vi "FLOM Pump Flow Write SubVI - standalone.vi"(0 "Write to Pump 1?":bool=TRUE, 1 "Write to Pump 2?":bool=TRUE, 2 "Mode":string(combo)="Continuous Flow", 3 "Edit Values, or Run Flow?\n(Only for Continuous Flow)":string(combo)="Run/Stop", 4 "Stop   Start":bool, 5 "Pump 1 Flow Rate (uL/min)":dbl=3000.0 min=0.0 max=9900.0 step=1.0, 6 "Stop   Start 2":bool, 7 "error in (no error) 2":errorcluster, 8 "Pump 2 Flow Rate (uL/min)":dbl=4000.0 min=0.0 max=9900.0 step=1.0, 9 "Data Cluster In":T1={"Flom Pump 1 Flow Rate"=0.0, "Script Running"=FALSE, "Unistat Set Temp"=0, "Flom Pump 2 Flow Rate"=0.0, "Flom Pump 1 Running"=FALSE, "Flom Pump 2 Running"=FALSE, "Unistat Running"=FALSE, "Line 1 Flow"=0.0, "Line 2 Flow"=0.0, "Product Temp"=0.0, "Product Flow"=0.0, "HEF Inlet"=0.0, "HEF Outlet"=0.0, "Line 1 Pressure"=0.0, "Line 2 Pressure"=0.0, "Line 3 Pressure"=0.0, "Pump 1 Pressure"=0.0, "Pump 2 Pressure"=0.0, "Number of Steps"=0.0, "Current Step Number"=0.0, "Pump 2 Flow Increment"=0.0, "Step Temp Increment"=0.0, "Step Function Start Time"=0.0, "Pump 2"=FALSE, "Pump 1"=TRUE, "Step Down?"=FALSE, "Number of Cycles"=0.0, "Pump 1 Initial Flow Rate"=0.0, "Pump 2 Initial Flow Rate"=0.0, "Initial Temperature"=0.0, "Step End Time"=0.0, "Pump 1 Current Step Flow"=0.0, "Pump 2 Current Step Flow"=0.0, "Current Step Temp"=0, "Time in each Step"=0.0, "Current Cycle Number"=0.0, "Turn off Temp after Step Flow?"=FALSE, "Internal Temp"=0.0, "Selected Path"=path "", "Excel Row Written"=0, "Counter at constant temp"=0.0, "Temp at Equilibrium"=FALSE, "Temp Equil Counter"=0.0, "Custom Step"=[{"Temp / C"=2, "Time / s"=0, "Flow 2 mL/m"=0.0, "Flow 1 mL/m"=0.0}, {"Temp / C"=2, "Time / s"=20, "Flow 2 mL/m"=0.0, "Flow 1 mL/m"=0.0}, {"Temp / C"=2, "Time / s"=100, "Flow 2 mL/m"=0.0, "Flow 1 mL/m"=0.0}, {"Temp / C"=2, "Time / s"=0, "Flow 2 mL/m"=0.0, "Flow 1 mL/m"=0.0}, {"Temp / C"=2, "Time / s"=90, "Flow 2 mL/m"=0.0, "Flow 1 mL/m"=0.0}, {"Temp / C"=2, "Time / s"=15, "Flow 2 mL/m"=0.0, "Flow 1 mL/m"=0.0}, {"Temp / C"=2, "Time / s"=0, "Flow 2 mL/m"=0.0, "Flow 1 mL/m"=0.0}, {"Temp / C"=2, "Time / s"=75, "Flow 2 mL/m"=0.0, "Flow 1 mL/m"=0.0}, {"Temp / C"=2, "Time / s"=2, "Flow 2 mL/m"=0.0, "Flow 1 mL/m"=0.0}], "Custom Step Number"=0.0, "Current Step t=0?"=FALSE, "Write to File"=FALSE, "Global Initialization Variables"={"Reactor Pressure Hard Upper Limit (bar)"=10.0, "Temp Hard Upper Limit (C)"=80.0, "Temp Hard Lower Limit (C)"=0.0, "Pump Minimum Flow (mL/min)"=0.0, "Pump Maximum Flow (mL/min)"=9.9, "Pump Interval (mL/min)"=0.001, "Temp Interval (C)"=0.1, "Flow Path Volume (mL)"=0.0}, "Error Message"="", "Program Error"=FALSE, "Pump Error"=FALSE, "Hardware Alert"=FALSE, "Comment"="", "Room Temp"=0.0, "VISA Resources"={"Flow VISA"="COM43", "Temp VISA"="COM43", "Flow VISA 1"="COM43", "Flow VISA 2"="COM43", "Flow VISA 3"="COM43", "Pressure VISA"="COM43", "Series IA VISA"="", "Series IB VISA"="", "Flow VISA 4"=""}, "Write Error"=FALSE, "Ports 1-5"=[FALSE, FALSE, FALSE, FALSE, FALSE, FALSE, FALSE, FALSE], "Pump 1 Flow Increment"=0.0, "Send to Product?"=FALSE, "Raman Spectrum Path"=path "", "Raman Spectrum Count"=0.0, "% Yield"=0.0, "Raman File Name"="", "New Spectrum?"=FALSE, "Last Spectrum Collected"=timestamp(0 s since 1904-01-01), "Line 4 Pressure"=0.0, "Series IA Pump Running"=FALSE, "Series IB Pump Running"=FALSE, "Series IA Pump Flow Rate"=0.0, "Series IB Pump Flow Rate"=0.0, "Line 3 Flow"=0.0, "Line 4 Flow"=0.0, "Series IA Pump Pressure"=0.0, "Series IB Pump Pressure"=0.0, "Flow Meter Cal Values"={"Flow Meter 2 Span Flow Rate"=10.0, "Flow Meter 1 Min Counts"=0.0, "Flow Meter 1 Max Counts"=9.9, "Flow Meter 1 Span Flow Rate"=0.01, "Flow Meter 2 Min Counts"=0.1, "Flow Meter 2 Max Counts"=0.0, "Flow Meter 4 Span Flow Rate"=10.0, "Flow Meter 3 Min Counts"=0.0, "Flow Meter 3 Max Counts"=9.9, "Flow Meter 3 Span Flow Rate"=0.01, "Flow Meter 4 Min Counts"=0.1, "Flow Meter 4 Max Counts"=0.0}, "Raman Exp?"=FALSE} {"Global Initialization Variables"."Reactor Pressure Hard Upper Limit (bar)" min=0.0 max=100.0 step=1.0}, 10 "Mode 2":string(combo)="Continuous Flow", 12 "Edit Values, or Run Flow?\n(Only for Continuous Flow) 2":string(combo)="Run/Stop", 15 "VISA resource":refnum<visa-resource-name>="COM8") -> (20 "Data Cluster Out":T1={"Flom Pump 1 Flow Rate"=0.0, "Script Running"=FALSE, "Unistat Set Temp"=0, "Flom Pump 2 Flow Rate"=0.0, "Flom Pump 1 Running"=FALSE, "Flom Pump 2 Running"=FALSE, "Unistat Running"=FALSE, "Line 1 Flow"=0.0, "Line 2 Flow"=0.0, "Product Temp"=0.0, "Product Flow"=0.0, "HEF Inlet"=0.0, "HEF Outlet"=0.0, "Line 1 Pressure"=0.0, "Line 2 Pressure"=0.0, "Line 3 Pressure"=0.0, "Pump 1 Pressure"=0.0, "Pump 2 Pressure"=0.0, "Number of Steps"=0.0, "Current Step Number"=0.0, "Pump 2 Flow Increment"=0.0, "Step Temp Increment"=0.0, "Step Function Start Time"=0.0, "Pump 2"=FALSE, "Pump 1"=TRUE, "Step Down?"=FALSE, "Number of Cycles"=0.0, "Pump 1 Initial Flow Rate"=0.0, "Pump 2 Initial Flow Rate"=0.0, "Initial Temperature"=0.0, "Step End Time"=0.0, "Pump 1 Current Step Flow"=0.0, "Pump 2 Current Step Flow"=0.0, "Current Step Temp"=0, "Time in each Step"=0.0, "Current Cycle Number"=0.0, "Turn off Temp after Step Flow?"=FALSE, "Internal Temp"=0.0, "Selected Path"=path "", "Excel Row Written"=0, "Counter at constant temp"=0.0, "Temp at Equilibrium"=FALSE, "Temp Equil Counter"=0.0, "Custom Step"=[{"Temp / C"=2, "Time / s"=0, "Flow 2 mL/m"=0.0, "Flow 1 mL/m"=0.0}, {"Temp / C"=2, "Time / s"=20, "Flow 2 mL/m"=0.0, "Flow 1 mL/m"=0.0}, {"Temp / C"=2, "Time / s"=100, "Flow 2 mL/m"=0.0, "Flow 1 mL/m"=0.0}, {"Temp / C"=2, "Time / s"=0, "Flow 2 mL/m"=0.0, "Flow 1 mL/m"=0.0}, {"Temp / C"=2, "Time / s"=90, "Flow 2 mL/m"=0.0, "Flow 1 mL/m"=0.0}, {"Temp / C"=2, "Time / s"=15, "Flow 2 mL/m"=0.0, "Flow 1 mL/m"=0.0}, {"Temp / C"=2, "Time / s"=0, "Flow 2 mL/m"=0.0, "Flow 1 mL/m"=0.0}, {"Temp / C"=2, "Time / s"=75, "Flow 2 mL/m"=0.0, "Flow 1 mL/m"=0.0}, {"Temp / C"=2, "Time / s"=2, "Flow 2 mL/m"=0.0, "Flow 1 mL/m"=0.0}], "Custom Step Number"=0.0, "Current Step t=0?"=FALSE, "Write to File"=FALSE, "Global Initialization Variables"={"Reactor Pressure Hard Upper Limit (bar)"=10.0, "Temp Hard Upper Limit (C)"=80.0, "Temp Hard Lower Limit (C)"=0.0, "Pump Minimum Flow (mL/min)"=0.0, "Pump Maximum Flow (mL/min)"=9.9, "Pump Interval (mL/min)"=0.001, "Temp Interval (C)"=0.1, "Flow Path Volume (mL)"=0.0}, "Error Message"="", "Program Error"=FALSE, "Pump Error"=FALSE, "Hardware Alert"=TRUE, "Comment"="", "Room Temp"=0.0, "VISA Resources"={"Flow VISA"="COM43", "Temp VISA"="COM43", "Flow VISA 1"="COM43", "Flow VISA 2"="COM43", "Flow VISA 3"="COM43", "Pressure VISA"="COM43", "Series IA VISA"="", "Series IB VISA"="", "Flow VISA 4"=""}, "Write Error"=FALSE, "Ports 1-5"=[FALSE, FALSE, FALSE, FALSE, FALSE, FALSE, FALSE, FALSE], "Pump 1 Flow Increment"=0.0, "Send to Product?"=FALSE, "Raman Spectrum Path"=path "", "Raman Spectrum Count"=0.0, "% Yield"=0.0, "Raman File Name"="", "New Spectrum?"=FALSE, "Last Spectrum Collected"=timestamp(0 s since 1904-01-01), "Line 4 Pressure"=0.0, "Series IA Pump Running"=FALSE, "Series IB Pump Running"=FALSE, "Series IA Pump Flow Rate"=0.0, "Series IB Pump Flow Rate"=0.0, "Line 3 Flow"=0.0, "Line 4 Flow"=0.0, "Series IA Pump Pressure"=0.0, "Series IB Pump Pressure"=0.0, "Flow Meter Cal Values"={"Flow Meter 2 Span Flow Rate"=10.0, "Flow Meter 1 Min Counts"=0.0, "Flow Meter 1 Max Counts"=9.9, "Flow Meter 1 Span Flow Rate"=0.01, "Flow Meter 2 Min Counts"=0.1, "Flow Meter 2 Max Counts"=0.0, "Flow Meter 4 Span Flow Rate"=10.0, "Flow Meter 3 Min Counts"=0.0, "Flow Meter 3 Max Counts"=9.9, "Flow Meter 3 Span Flow Rate"=0.01, "Flow Meter 4 Min Counts"=0.1, "Flow Meter 4 Max Counts"=0.0}, "Raman Exp?"=FALSE} {"Global Initialization Variables"."Reactor Pressure Hard Upper Limit (bar)" min=0.0 max=100.0 step=1.0}, 27 "Error Out":T2)   [LabVIEW 2015]
doc: "Written 12/2010 by Michael Roberto for control and monitoring of Flom high pressure liquid chromatography (HPLC) pumps.\n\nThis VI's purpose is to control the HPLC pumps, in conjunctiton with monitoring pressure and temperature in the reactor, and controlling the temperature via a heating system (yet to be integrated). To do this, the user first chooses the COM port in the VISA resource name box. Then pump number (set up seperately on the pump) is chosen. The user then chooses what kind of interaction they wish to perform with the pump: Continuous Flow, Step Flow, Status, or Reset. Discussion will focus mostly on Continuous and Step Flow commands.\n\nTo execute any command, the EXECUTE button must be pressed, to ensure that the commands are all set and that the pump receives the command only once.\n\nWhen using Continuous Flow, only use the drop down box labeled \"Only for Continuous Flow.\" Using the other boxes or numeric indicators when they're not specifically queried will not cause an error, but it's easier to understand when they're clear or, in the case of step number or time for continuous flow, zero. The flow rate for continuous flow is set seperately from the run/stop command. To edit the flow rate, choose \"edit\" from the drop-down menu and enter a flow rate in the Flow Rate box. Press the EXECUTE button to send the command to the pump. To begin flow, choose \"Start/Stop\" from the drop-down box, and set the switch into the \"Start\" position, and press the EXECUTE button. To stop, switch to Stop and press EXECUTE.\nIn continuous flow, flow rate can be changed while the pump is flowing. Same as before, choose \"edit,\" enter the flow rate, and press EXECUTE.\n\nStep mode is more complicated to run, as flow rates need to be established for each step separately, and the initial flow rate must stipulate how many steps will be executed. I hope to write a VI in the future that, when given a command such as \"20 steps, 0.1 ul/min increments, for 20 minutes,\" will go through and perform these itself, but for now they each have to be performed separately.\n\nGeneric Step Instructions: \nFirst, set up an initial flow rate by choosing such in the drop down menu. It's *important* that you dictate how many steps will be in the program as well. It must be chosen before you hit EXECUTE when setting the initial flow rate.\nSecond, you must define the flow rate and time and step method (linear vs. step) for each step, in the 'configure step' drop down menu. So you would set the step at \"1\", flow rate at the desired flow, and for the desired time length, then press EXECUTE. Then change all those variables again for the 2nd step, and so on. The pump will not recognize commands if you exceed the number of steps dictated in the initial flow rate.\nThird, you run the initial flow rate, by choosing so from the drop down menu and pressing EXECUTE when the switch is in the Start position\nFourth, run the step program.\nAfter the Step Program has finished, the pump will return to the initial flow rate, and will not turn off until you switch to \"Stop\" while in the \"Run initial flow rate\" drop down and hitting EXECUTE."
uses:
  --Controls and TypeDefs--/Control_LDH.ctl
  <vilib>/Instr/_visa.llb/VISA Configure Serial Port (Instr).vi
panel:
  in  "Step   Linear 2":bool
  in  "Step Flow Commands \n(Only For Step Flow) 2":string(combo)
  in  "Time (.01 mins) 2":i32 min=0 max=9999 step=1
  in  "Step # 2":i32 min=0 max=49 step=1
  in  "Setup Commands\n(Only for Setup) 2":string(combo)
  in  "Request Commands\n(Only for Status) 2":string(combo)
  in  "Step   Linear":bool
  out "String to Write to Pump 2":string="P2,G1,0"
  in  "bytes to read 2":u32=40
  out "actual bytes read 2":u32=9
  out "P2 Flowing?":bool
  out "Last message received from Pump 2":string="Pump 2 message, 10:06:19 AM:\nProgram Error: Prohibited command (conflicting operation command)"
  out "Status of Pump 2":string
  out "P1 Flowing?":bool
  out "Last message received from Pump 1":string="Pump 1 message, 10:06:19 AM:\nProgram Error: Prohibited command (conflicting operation command)"
  in  "Step Flow Commands \n(Only For Step Flow)":string(combo)
  in  "Time (.01 mins)":i32 min=0 max=9999 step=1
  in  "Step #":i32 min=0 max=49 step=1
  in  "Setup Commands\n(Only for Setup)":string(combo)
  in  "Request Commands\n(Only for Status)":string(combo)
  out "String to Write to Pump 1":string="P1,G1,0"
  out "actual bytes read":u32=8
  in  "bytes to read":u32=40
  out "Status of Pump 1":string
  # "Flom Pump Control VI.  Continuously queries status of pump, writes to pump with \"EXECUTE\" button press."
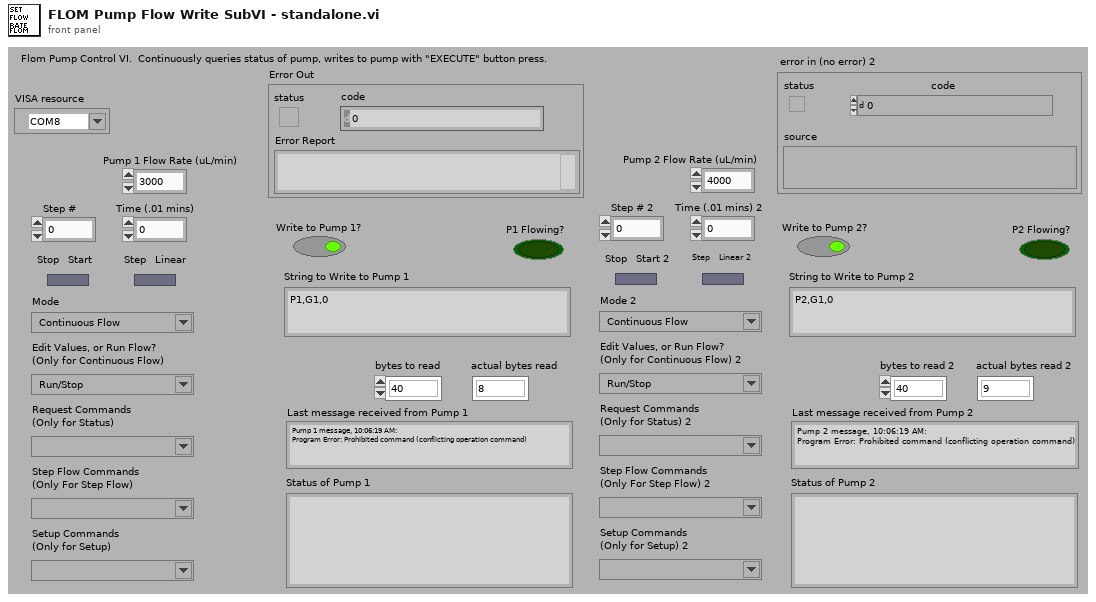
[diagram p1: front panel]
types:
  T1 = typedef "Control_LDH.ctl" = cluster{"Flom Pump 1 Flow Rate":dbl, "Script Running":bool, "Unistat Set Temp":i32, "Flom Pump 2 Flow Rate":dbl, "Flom Pump 1 Running":bool, "Flom Pump 2 Running":bool, "Unistat Running":bool, "Line 1 Flow":dbl, "Line 2 Flow":dbl, "Product Temp":dbl, "Product Flow":dbl, "HEF Inlet":dbl, "HEF Outlet":dbl, "Line 1 Pressure":dbl, "Line 2 Pressure":dbl, "Line 3 Pressure":dbl, "Pump 1 Pressure":dbl, "Pump 2 Pressure":dbl, "Number of Steps":dbl, "Current Step Number":dbl, "Pump 2 Flow Increment":dbl, "Step Temp Increment":dbl, "Step Function Start Time":dbl, "Pump 2":bool, "Pump 1":bool, "Step Down?":bool, "Number of Cycles":dbl, "Pump 1 Initial Flow Rate":dbl, "Pump 2 Initial Flow Rate":dbl, "Initial Temperature":dbl, "Step End Time":dbl, "Pump 1 Current Step Flow":dbl, "Pump 2 Current Step Flow":dbl, "Current Step Temp":i32, "Time in each Step":dbl, "Current Cycle Number":dbl, "Turn off Temp after Step Flow?":bool, "Internal Temp":dbl, "Selected Path":path, "Excel Row Written":i32, "Counter at constant temp":dbl, "Temp at Equilibrium":bool, "Temp Equil Counter":dbl, "Custom Step":cluster{"Temp / C":u16, "Time / s":i32, "Flow 2 mL/m":dbl, "Flow 1 mL/m":dbl}[], "Custom Step Number":dbl, "Current Step t=0?":bool, "Write to File":bool, "Global Initialization Variables":cluster{"Reactor Pressure Hard Upper Limit (bar)":dbl, "Temp Hard Upper Limit (C)":dbl, "Temp Hard Lower Limit (C)":dbl, "Pump Minimum Flow (mL/min)":dbl, "Pump Maximum Flow (mL/min)":dbl, "Pump Interval (mL/min)":dbl, "Temp Interval (C)":dbl, "Flow Path Volume (mL)":dbl}, "Error Message":string, "Program Error":bool, "Pump Error":bool, "Hardware Alert":bool, "Comment":string, "Room Temp":dbl, "VISA Resources":cluster{"Flow VISA":refnum<visa-resource-name>, "Temp VISA":refnum<visa-resource-name>, "Flow VISA 1":refnum<visa-resource-name>, "Flow VISA 2":refnum<visa-resource-name>, "Flow VISA 3":refnum<visa-resource-name>, "Pressure VISA":refnum<visa-resource-name>, "Series IA VISA":refnum<visa-resource-name>, "Series IB VISA":refnum<visa-resource-name>, "Flow VISA 4":refnum<visa-resource-name>}, "Write Error":bool, "Ports 1-5":bool[], "Pump 1 Flow Increment":dbl, "Send to Product?":bool, "Raman Spectrum Path":path, "Raman Spectrum Count":dbl, "% Yield":dbl, "Raman File Name":string, "New Spectrum?":bool, "Last Spectrum Collected":timestamp, "Line 4 Pressure":dbl, "Series IA Pump Running":bool, "Series IB Pump Running":bool, "Series IA Pump Flow Rate":dbl, "Series IB Pump Flow Rate":dbl, "Line 3 Flow":dbl, "Line 4 Flow":dbl, "Series IA Pump Pressure":dbl, "Series IB Pump Pressure":dbl, "Flow Meter Cal Values":cluster{"Flow Meter 2 Span Flow Rate":dbl, "Flow Meter 1 Min Counts":dbl, "Flow Meter 1 Max Counts":dbl, "Flow Meter 1 Span Flow Rate":dbl, "Flow Meter 2 Min Counts":dbl, "Flow Meter 2 Max Counts":dbl, "Flow Meter 4 Span Flow Rate":dbl, "Flow Meter 3 Min Counts":dbl, "Flow Meter 3 Max Counts":dbl, "Flow Meter 3 Span Flow Rate":dbl, "Flow Meter 4 Min Counts":dbl, "Flow Meter 4 Max Counts":dbl}, "Raman Exp?":bool}
  T2 = cluster{"status":bool, "code":i32, "Error Report":string}
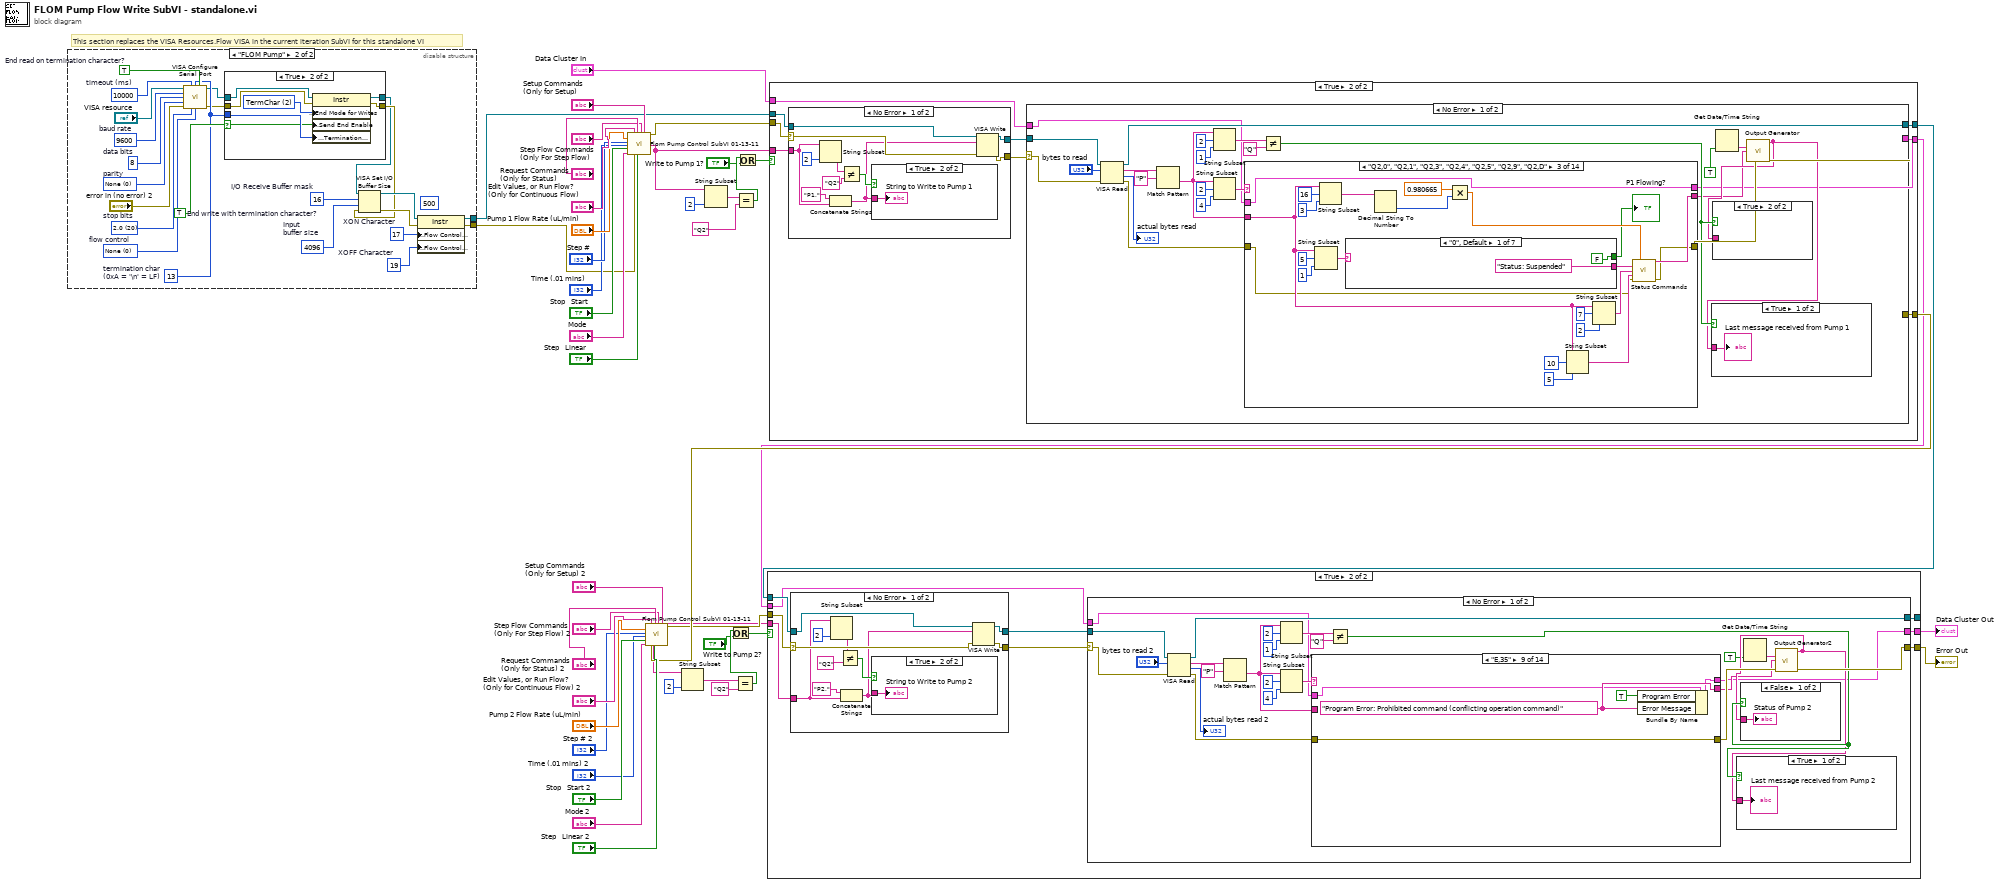
[diagram p0: block diagram]
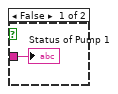
[diagram p5: hidden frame]
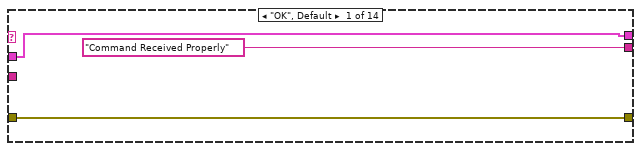
[diagram p7: hidden frame]
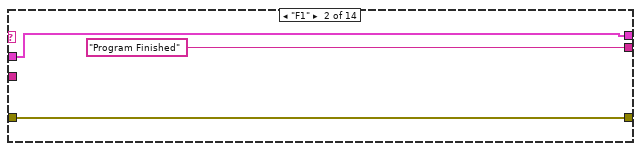
[diagram p8: hidden frame]
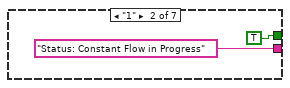
[diagram p9: hidden frame]
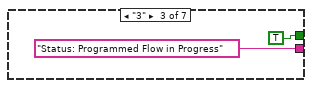
[diagram p10: hidden frame]
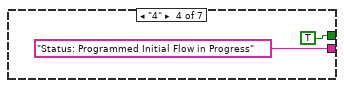
[diagram p11: hidden frame]
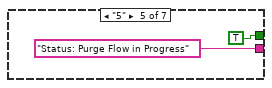
[diagram p12: hidden frame]
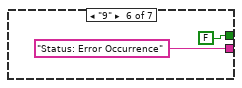
[diagram p13: hidden frame]
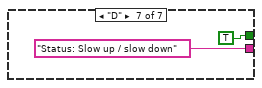
[diagram p14: hidden frame]
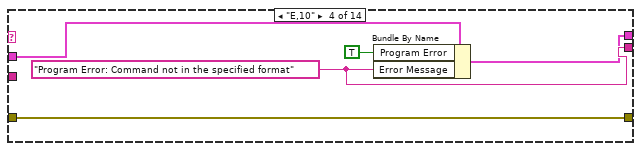
[diagram p15: hidden frame]
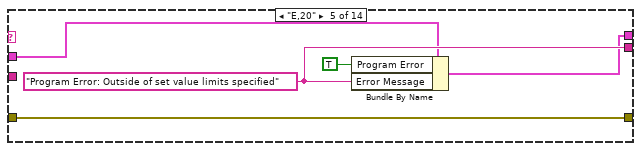
[diagram p16: hidden frame]
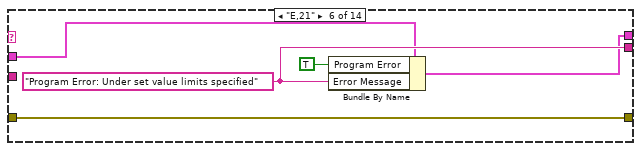
[diagram p17: hidden frame]
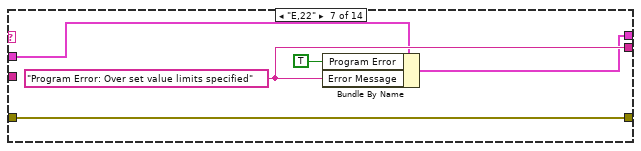
[diagram p18: hidden frame]
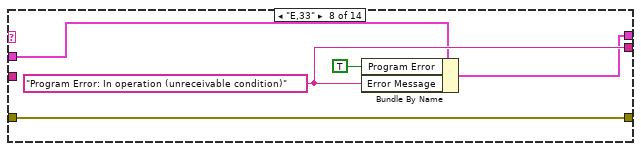
[diagram p19: hidden frame]
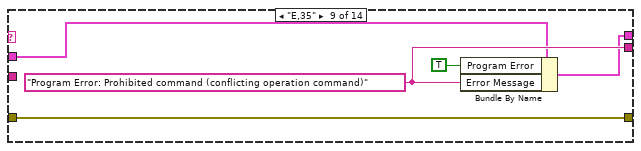
[diagram p20: hidden frame]
diagram:
  # "This section replaces the VISA Resources.Flow VISA in the current iteration SubVI for this standalone VI"
  n1 = disable-structure shown="\"FLOM Pump\"" {
    disable-tunnel: [_ w47] -> w2
    disable-tunnel: [_ w46] -> w1
    frame condition #0 {
    }
    frame condition #1 (active) {
      (unwired) 500
      w60 = u32 4096  # Input buffer size
      w53 = u8 19  # XOFF Character
      w54 = u8 17  # XON Character
      w63 = u32 10000  # timeout (ms)
      w62 = TRUE  # End read on termination character?
      w59 = TRUE  # End write with termination character?
      w58 = u8 13  # termination char (0xA = '\n' = LF)
      w57 = u16 0 items=["None"=0, "XON/XOFF"=1, "RTS/CTS"=2, "DTR/DSR"=4]  # flow control
      w64 = u16 20 items=["1.0"=10, "1.5"=15, "2.0"=20]  # stop bits
      w65 = u16 0 items=["None", "Odd", "Even", "Mark", "Space"]  # parity
      w52 = u16 8  # data bits
      w67 = u32 9600  # baud rate
      w61 = u16 16  # I/O Receive Buffer mask
      n2 = call-poly "VISA Configure Serial Port"("VISA resource name"="VISA resource", "timeout (10sec)"=w63, "termination char\n(0xA = '\\n' = LF)"=w58, "Enable Termination\nChar (T)"=w62, "baud rate (9600)"=w67, "data bits (8)"=w52, "parity (0:none)"=w65, "error in (no error)"="error in (no error) 2", "stop bits (10: 1 bit)"=w64, "flow control (0:none)"=w57) -> ("VISA resource name out"=w48:refnum<visa-resource-name>, "error out"=w51:errorcluster)  [unwired: 4 out]
      n3 = case shown="True" w59 {
        selector: w59 -> [_ w70]
        tunnel: w48 -> [w68 w76]
        tunnel: w51 -> [w69 w75]
        tunnel: [w68 w74] -> w49
        tunnel: [w69 w73] -> w50
        tunnel: w58 -> [_ w71]
        frame False {
        }
        frame True {
          w72 = u16 2 items=["None", "LastBit", "TermChar", "Break"] ("Serial Settings:Serial End Mode for Writes")
          n4 = property class="Instr"(reference=w76, error in=w75, "Serial Settings:End Mode for Writes"=w72, "Message Based Settings:Send End Enable"=w70, "Message Based Settings:Termination Character"=w71) -> (reference out=w74:refnum<visa-resource-name>, error out=w73:errorcluster)
        }
      }
      n5 = VISA Set I/O Buffer Size(VISA resource name=w49, mask (16)=w61, size (4096)=w60, error in (no error)=w50) -> (VISA resource name out=w56:refnum<visa-resource-name>, error out=w55:errorcluster)
      n6 = property class="Instr"(reference=w56, error in=w55, "Serial Settings:Flow Control XON Character"=w54, "Serial Settings:Flow Control XOFF Character"=w53) -> (reference out=w46:refnum<visa-resource-name>, error out=w47:errorcluster)
    }
  }
  n7 = call "Flom Pump Control SubVI 01-13-11.vi"("Flow Rate (uL)"="Pump 1 Flow Rate (uL/min)", "Step #"="Step #", "Time (.01 mins)"="Time (.01 mins)", "Stop   Start"="Stop   Start", "Mode"="Mode", "Edit Values, or Run Flow?\n(Only for Continuous Flow)"="Edit Values, or Run Flow?\n(Only for Continuous Flow)", "error in (no error)"=w2, "Request Commands\n(Only for Status)"="Request Commands\n(Only for Status)", "Step Linear"="Step   Linear", "Step Flow Commands \n(Only For Step Flow)"="Step Flow Commands \n(Only For Step Flow)", "Setup Commands\n(Only for Setup)"="Setup Commands\n(Only for Setup)") -> ("error out"=w4:errorcluster, "String"=w40:string)  [unwired: 1 in, 6 out]
  n8 = String Subset(string=w40, length (rest)=2) -> (substring=w42:string)  [unwired: 1 out]
  n9 = Equal?(x=w42, y="Q2") -> (x = y?=w39:bool)
  n10 = Or(x=w39, y="Write to Pump 1?") -> (x .or. y?=w37:bool)
  n11 = case shown="True" w37 {
    tunnel: w1 -> [w79 w86]
    tunnel: w4 -> [w78 w85]
    tunnel: [w79 w84] -> w44
    tunnel: [w78 w83] -> w10
    tunnel: w40 -> [_ w82]
    tunnel: "Data Cluster In" -> [w77 w81]
    tunnel: [w77 w80] -> w7
    frame False {
    }
    frame True {
      n12 = case shown="No Error" w85 {
        selector: w85 -> [w223 w229]
        tunnel: [w226 w228] -> w88
        tunnel: [w225 w229] -> w87
        tunnel: w86 -> [w224 w228]
        tunnel: w82 -> [w217 _]
        frame No Error {
          n13 = String Subset(string=w217, length (rest)=2) -> (substring=w220:string)  [unwired: 1 out]
          n14 = Concatenate Strings("P1,", w217) -> (w216:string)
          n15 = Not Equal?(x=w220, y="Q2") -> (x != y?=w218:bool)
          n16 = case shown="True" w218 {
            tunnel: w216 -> [_ w227]
            frame False {
            }
            frame True {
              "String to Write to Pump 1" <- w227
            }
          }
          n17 = VISA Write(VISA resource name=w224, write buffer=w216, error in (no error)=w223) -> (VISA resource name out=w226:refnum<visa-resource-name>, error out=w225:errorcluster)  [unwired: 1 out]
        }
        frame Error {
        }
      }
      n18 = case "Read bytes from port." shown="No Error" w87 {
        selector: w87 -> [w110 w214]
        tunnel: [w97 w214] -> w83
        tunnel: [w113 w215] -> w84
        tunnel: w88 -> [w111 w215]
        tunnel: w81 -> [w90 w213]
        tunnel: [w89 w213] -> w80
        frame No Error {
          n19 = VISA Read(VISA resource name=w111, byte count="bytes to read", error in (no error)=w110) -> (VISA resource name out=w113:refnum<visa-resource-name>, read buffer=w104:string, return count=→"actual bytes read":u32, error out=w99:errorcluster)
          n20 = Match Pattern(string=w104, regular expression="P") -> (after substring=w96:string)  [unwired: 4 out]
          n21 = String Subset(string=w96, offset (0)=2, length (rest)=1) -> (substring=w101:string)
          n22 = String Subset(string=w96, offset (0)=2, length (rest)=4) -> (substring=w108:string)
          n23 = case shown="\"Q2,0\", \"Q2,1\", \"Q2,3\", \"Q2,4\", \"Q2,5\", \"Q2,9\", \"Q2,D\"" w108 {
            tunnel: ["Command Received Properly" "Program Finished" w128 w159 w165 w170 w175 w180 w185 w190 w195 w200 w205 w210] -> w91
            tunnel: w96 -> [_ _ w126 _ _ _ _ _ _ _ _ _ _ _]
            tunnel: w99 -> [w117 w120 w125 w162 w167 w172 w177 w182 w187 w192 w197 w202 w207 w212]
            tunnel: [w117 w120 w124 w162 w167 w172 w177 w182 w187 w192 w197 w202 w207 w212] -> w98
            tunnel: w90 -> [w116 w119 w122 w161 w164 w168 w174 w179 w184 w189 w194 w199 w204 w209]
            tunnel: [w116 w119 w122 w158 w163 w169 w173 w178 w183 w188 w193 w198 w203 w208] -> w89
            frame "OK", Default {
            }
            frame "F1" {
            }
            frame "Q2,0", "Q2,1", "Q2,3", "Q2,4", "Q2,5", "Q2,9", "Q2,D" {
              n24 = String Subset(string=w126, offset (0)=5, length (rest)=1) -> (substring=w127:string)
              n25 = String Subset(string=w126, offset (0)=16, length (rest)=3) -> (substring=w135:string)
              n26 = case shown="\"0\", Default" w127 {
                tunnel: ["Status: Suspended" "Status: Constant Flow in Progress" "Status: Programmed Flow in Progress" "Status: Programmed Initial Flow in Progress" "Status: Purge Flow in Progress" "Status: Error Occurrence" "Status: Slow up / slow down"] -> w132
                tunnel: [FALSE TRUE TRUE TRUE TRUE FALSE TRUE] -> w123
                frame "0", Default {
                }
                frame "1" {
                }
                frame "3" {
                }
                frame "4" {
                }
                frame "5" {
                }
                frame "9" {
                }
                frame "D" {
                }
              }
              "P1 Flowing?" <- w123
              n27 = Decimal String To Number(string=w135) -> (number=w134:i32)  [unwired: 3 out]
              n28 = Multiply(x=0.980665, y=w134) -> (x*y=w129:dbl)
              n29 = String Subset(string=w126, offset (0)=10, length (rest)=5) -> (substring=w130:string)
              n30 = String Subset(string=w126, offset (0)=7, length (rest)=2) -> (substring=w131:string)
              n31 = call "Status Commands"("press"=w129, "Status"=w132, "step num"=w131, "flow"=w130, "error in (no error)"=w125) -> ("Result"=w128:string, "error out"=w124:errorcluster)  [unwired: 1 in, 8 out]
            }
            frame "E,10" {
              w159 = "Program Error: Command not in the specified format"
              n32 = Bundle By Name(cluster=w161, "Program Error"=TRUE, "Error Message"=w159) -> (w158:T1)
            }
            frame "E,20" {
              w165 = "Program Error: Outside of set value limits specified"
              n33 = Bundle By Name(cluster=w164, "Program Error"=TRUE, "Error Message"=w165) -> (w163:T1)
            }
            frame "E,21" {
              w170 = "Program Error: Under set value limits specified"
              n34 = Bundle By Name(cluster=w168, "Program Error"=TRUE, "Error Message"=w170) -> (w169:T1)
            }
            frame "E,22" {
              w175 = "Program Error: Over set value limits specified"
              n35 = Bundle By Name(cluster=w174, "Program Error"=TRUE, "Error Message"=w175) -> (w173:T1)
            }
            frame "E,33" {
              w180 = "Program Error: In operation (unreceivable condition)"
              n36 = Bundle By Name(cluster=w179, "Program Error"=TRUE, "Error Message"=w180) -> (w178:T1)
            }
            frame "E,35" {
              w185 = "Program Error: Prohibited command (conflicting operation command)"
              n37 = Bundle By Name(cluster=w184, "Program Error"=TRUE, "Error Message"=w185) -> (w183:T1)
            }
            frame "E,52" {
              w190 = "Program Error: Error due to unconnected subordinate pumps (CTS error)"
              n38 = Bundle By Name(cluster=w189, "Program Error"=TRUE, "Error Message"=w190) -> (w188:T1)
            }
            frame "E,61" {
              w195 = "Pump Error: Error after the upper pressure limit is exceeded"
              n39 = Bundle By Name(cluster=w194, "Pump Error"=TRUE, "Error Message"=w195) -> (w193:T1)
            }
            frame "E,62" {
              w200 = "Pump Error: Error after the lower pressure limit is exceeded"
              n40 = Bundle By Name(cluster=w199, "Pump Error"=TRUE, "Error Message"=w200) -> (w198:T1)
            }
            frame "E,63" {
              w205 = "Pump Error: Check-valve error"
              n41 = Bundle By Name(cluster=w204, "Pump Error"=TRUE, "Error Message"=w205) -> (w203:T1)
            }
            frame "E,64" {
              w210 = "Pump Error: Irregular Rotation Error"
              n42 = Bundle By Name(cluster=w209, "Pump Error"=TRUE, "Error Message"=w210) -> (w208:T1)
            }
          }
          n43 = Not Equal?(x=w101, y="Q") -> (x != y?=w95:bool)
          n44 = Get Date/Time String(want seconds? (F)=TRUE) -> (time string=w92:string)  [unwired: 3 out]
          n45 = call "Output Generator"("Time"=w92, "Error Output"=w91, "error in (no error)"=w98) -> ("Result"=w94:string, "error out"=w97:errorcluster)  [unwired: 2 in, 9 out]
          n46 = case shown="True" w95 {
            tunnel: w94 -> [w115 _]
            frame True {
              "Last message received from Pump 1" <- w115
            }
            frame False {
            }
          }
          n47 = case shown="True" w95 {
            tunnel: w94 -> [w114 _]
            frame False {
              "Status of Pump 1" <- w114
            }
            frame True {
            }
          }
        }
        frame Error {
        }
      }
    }
  }
  n48 = call "Flom Pump Control SubVI 01-13-11.vi"("Flow Rate (uL)"="Pump 2 Flow Rate (uL/min)", "Step #"="Step # 2", "Time (.01 mins)"="Time (.01 mins) 2", "Stop   Start"="Stop   Start 2", "Mode"="Mode 2", "Edit Values, or Run Flow?\n(Only for Continuous Flow)"="Edit Values, or Run Flow?\n(Only for Continuous Flow) 2", "error in (no error)"=w10, "Request Commands\n(Only for Status)"="Request Commands\n(Only for Status) 2", "Step Linear"="Step   Linear 2", "Step Flow Commands \n(Only For Step Flow)"="Step Flow Commands \n(Only For Step Flow) 2", "Setup Commands\n(Only for Setup)"="Setup Commands\n(Only for Setup) 2") -> ("error out"=w9:errorcluster, "String"=w8:string)  [unwired: 1 in, 6 out]
  n49 = String Subset(string=w8, length (rest)=2) -> (substring=w35:string)  [unwired: 1 out]
  n50 = Equal?(x=w35, y="Q2") -> (x = y?=w33:bool)
  n51 = Or(x=w33, y="Write to Pump 2?") -> (x .or. y?=w31:bool)
  n52 = case shown="True" w31 {
    tunnel: [w231 w239] -> w3
    tunnel: [w232 w238] -> _
    tunnel: w44 -> [w232 w237]
    tunnel: w9 -> [w231 w236]
    tunnel: w8 -> [_ w235]
    tunnel: w7 -> [w230 w234]
    tunnel: [w230 w233] -> w6
    frame False {
    }
    frame True {
      n53 = case shown="No Error" w236 {
        selector: w236 -> [w249 w255]
        tunnel: [w252 w254] -> w241
        tunnel: [w251 w255] -> w240
        tunnel: w237 -> [w250 w254]
        tunnel: w235 -> [w242 _]
        frame No Error {
          n54 = String Subset(string=w242, length (rest)=2) -> (substring=w246:string)  [unwired: 1 out]
          n55 = Not Equal?(x=w246, y="Q2") -> (x != y?=w244:bool)
          n56 = Concatenate Strings("P2,", w242) -> (w243:string)
          n57 = case shown="True" w244 {
            tunnel: w243 -> [_ w253]
            frame False {
            }
            frame True {
              "String to Write to Pump 2" <- w253
            }
          }
          n58 = VISA Write(VISA resource name=w250, write buffer=w243, error in (no error)=w249) -> (VISA resource name out=w252:refnum<visa-resource-name>, error out=w251:errorcluster)  [unwired: 1 out]
        }
        frame Error {
        }
      }
      n59 = case "Read bytes from port." shown="No Error" w240 {
        selector: w240 -> [w277 w381]
        tunnel: [w264 w381] -> w239
        tunnel: [w280 w382] -> w238
        tunnel: w241 -> [w278 w382]
        tunnel: w234 -> [w257 w380]
        tunnel: [w256 w380] -> w233
        frame No Error {
          n60 = VISA Read(VISA resource name=w278, byte count="bytes to read 2", error in (no error)=w277) -> (VISA resource name out=w280:refnum<visa-resource-name>, read buffer=w271:string, return count=→"actual bytes read 2":u32, error out=w266:errorcluster)
          n61 = Match Pattern(string=w271, regular expression="P") -> (after substring=w263:string)  [unwired: 4 out]
          n62 = String Subset(string=w263, offset (0)=2, length (rest)=1) -> (substring=w268:string)
          n63 = String Subset(string=w263, offset (0)=2, length (rest)=4) -> (substring=w275:string)
          n64 = case shown="\"E,35\"" w275 {
            tunnel: ["Command Received Properly" "Program Finished" w295 w327 w332 w337 w341 w347 w352 w356 w360 w367 w372 w377] -> w258
            tunnel: w263 -> [_ _ w293 _ _ _ _ _ _ _ _ _ _ _]
            tunnel: w266 -> [w284 w287 w292 w329 w334 w339 w344 w349 w354 w359 w364 w369 w374 w379]
            tunnel: [w284 w287 w291 w329 w334 w339 w344 w349 w354 w359 w364 w369 w374 w379] -> w265
            tunnel: w257 -> [w283 w286 w289 w326 w331 w336 w342 w346 w351 w357 w362 w366 w371 w376]
            tunnel: [w283 w286 w289 w325 w330 w335 w340 w345 w350 w355 w361 w365 w370 w375] -> w256
            frame "OK", Default {
            }
            frame "F1" {
            }
            frame "Q2,0", "Q2,1", "Q2,3", "Q2,4", "Q2,5", "Q2,9", "Q2,D" {
              n65 = String Subset(string=w293, offset (0)=5, length (rest)=1) -> (substring=w294:string)
              n66 = String Subset(string=w293, offset (0)=16, length (rest)=3) -> (substring=w302:string)
              n67 = case shown="\"4\"" w294 {
                tunnel: ["Status: Suspended" "Status: Constant Flow in Progress" "Status: Programmed Flow in Progress" "Status: Programmed Initial Flow in Progress" "Status: Purge Flow in Progress" "Status: Error Occurrence" "Status: Slow up / slow down"] -> w299
                tunnel: [FALSE TRUE TRUE TRUE TRUE FALSE TRUE] -> w290
                frame "0", Default {
                }
                frame "1" {
                }
                frame "3" {
                }
                frame "4" {
                }
                frame "5" {
                }
                frame "9" {
                }
                frame "D" {
                }
              }
              "P2 Flowing?" <- w290
              n68 = Decimal String To Number(string=w302) -> (number=w301:i32)  [unwired: 3 out]
              n69 = String Subset(string=w293, offset (0)=10, length (rest)=5) -> (substring=w297:string)
              n70 = Multiply(x=0.980665, y=w301) -> (x*y=w296:dbl)
              n71 = String Subset(string=w293, offset (0)=7, length (rest)=2) -> (substring=w298:string)
              n72 = call "Status Commands2"("press"=w296, "Status"=w299, "step num"=w298, "flow"=w297, "error in (no error)"=w292) -> ("Result"=w295:string, "error out"=w291:errorcluster)  [unwired: 1 in, 8 out]
            }
            frame "E,10" {
              w327 = "Program Error: Command not in the specified format"
              n73 = Bundle By Name(cluster=w326, "Program Error"=TRUE, "Error Message"=w327) -> (w325:T1)
            }
            frame "E,20" {
              w332 = "Program Error: Outside of set value limits specified"
              n74 = Bundle By Name(cluster=w331, "Program Error"=TRUE, "Error Message"=w332) -> (w330:T1)
            }
            frame "E,21" {
              w337 = "Program Error: Under set value limits specified"
              n75 = Bundle By Name(cluster=w336, "Program Error"=TRUE, "Error Message"=w337) -> (w335:T1)
            }
            frame "E,22" {
              w341 = "Program Error: Over set value limits specified"
              n76 = Bundle By Name(cluster=w342, "Program Error"=TRUE, "Error Message"=w341) -> (w340:T1)
            }
            frame "E,33" {
              w347 = "Program Error: In operation (unreceivable condition)"
              n77 = Bundle By Name(cluster=w346, "Program Error"=TRUE, "Error Message"=w347) -> (w345:T1)
            }
            frame "E,35" {
              w352 = "Program Error: Prohibited command (conflicting operation command)"
              n78 = Bundle By Name(cluster=w351, "Program Error"=TRUE, "Error Message"=w352) -> (w350:T1)
            }
            frame "E,52" {
              w356 = "Program Error: Error due to unconnected subordinate pumps (CTS error)"
              n79 = Bundle By Name(cluster=w357, "Program Error"=TRUE, "Error Message"=w356) -> (w355:T1)
            }
            frame "E,61" {
              w360 = "Pump Error: Error after the upper pressure limit is exceeded"
              n80 = Bundle By Name(cluster=w362, "Pump Error"=TRUE, "Error Message"=w360) -> (w361:T1)
            }
            frame "E,62" {
              w367 = "Pump Error: Error after the lower pressure limit is exceeded"
              n81 = Bundle By Name(cluster=w366, "Pump Error"=TRUE, "Error Message"=w367) -> (w365:T1)
            }
            frame "E,63" {
              w372 = "Pump Error: Check-valve error"
              n82 = Bundle By Name(cluster=w371, "Pump Error"=TRUE, "Error Message"=w372) -> (w370:T1)
            }
            frame "E,64" {
              w377 = "Pump Error: Irregular Rotation Error"
              n83 = Bundle By Name(cluster=w376, "Pump Error"=TRUE, "Error Message"=w377) -> (w375:T1)
            }
          }
          n84 = Not Equal?(x=w268, y="Q") -> (x != y?=w262:bool)
          n85 = Get Date/Time String(want seconds? (F)=TRUE) -> (time string=w259:string)  [unwired: 3 out]
          n86 = call "Output Generator2"("Time"=w259, "Error Output"=w258, "error in (no error)"=w265) -> ("Result"=w261:string, "error out"=w264:errorcluster)  [unwired: 2 in, 9 out]
          n87 = case shown="True" w262 {
            tunnel: w261 -> [w282 _]
            frame True {
              "Last message received from Pump 2" <- w282
            }
            frame False {
            }
          }
          n88 = case shown="False" w262 {
            tunnel: w261 -> [w281 _]
            frame False {
              "Status of Pump 2" <- w281
            }
            frame True {
            }
          }
        }
        frame Error {
        }
      }
    }
  }
  "Error Out" <- w3
  "Data Cluster Out" <- w6
